vi "Plane_coordinates_Limit2Frame.vi"(7 "Frame Size":i32, 11 "Input Array":sgl[][](array[numeric])) -> (3 "XYZ Start":cluster{"X":sgl, "Y":sgl, "Z":sgl}[](array[cluster]))   [LabVIEW 2017]
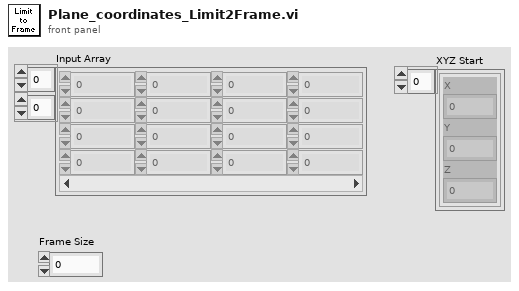
[diagram p1: front panel]
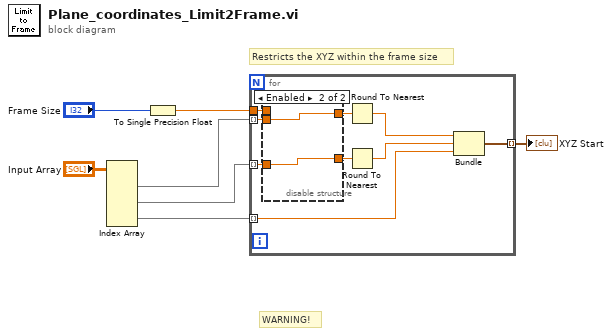
[diagram p0: block diagram]
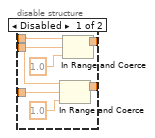
[diagram p2: hidden frame]
diagram:
  # "WARNING!"
  # "Restricts the XYZ within the frame size"
  n1 = Index Array(array="Input Array") -> (element #1=w4:sgl[], element #2=w6:sgl[], element #3=w3:sgl[])  [unwired: 6 in]
  n2 = To Single Precision Float(number="Frame Size") -> (single precision float=w1:sgl)
  n3 = for {
    tunnel: w1 -> [w13]
    tunnel: w6 -> [w15] mode=indexing
    tunnel: w4 -> [w12] mode=indexing
    tunnel: w3 -> [w9] mode=indexing
    tunnel: [w8] -> w2 mode=indexing
    n4 = disable-structure shown="Enabled" {
      disable-tunnel: [w22 w24] -> w16
      disable-tunnel: w15 -> [w21 w24]
      disable-tunnel: [w20 w25] -> w14
      disable-tunnel: w13 -> [w18 _]
      disable-tunnel: w12 -> [w17 w25]
      frame Disabled {
        n5 = In Range and Coerce(upper limit=w18, x=w21, lower limit=sgl 1.0) -> (coerced(x)=w22:sgl)  [unwired: 1 out]
        n6 = In Range and Coerce(upper limit=w18, x=w17, lower limit=sgl 1.0) -> (coerced(x)=w20:sgl)  [unwired: 1 out]
      }
      frame Enabled {
      }
    }
    n7 = Round To Nearest(number=w14) -> (nearest integer value=w11:sgl)
    n8 = Round To Nearest(number=w16) -> (nearest integer value=w10:sgl)
    n9 = Bundle(w11, w10, w9) -> (w8:cluster{sgl, sgl, sgl})  [unwired: 1 in]
  }
  "XYZ Start" <- w2
